vi "read_params.vi"(8 "error in (no error)":errorcluster caption="entrée d'erreur (pas d'erreur)", 11 "KMeans en entrée":refnum<class "KMeans.lvclass">) -> (0 "error out":errorcluster caption="sortie d'erreur", 2 "params":T1={"n_clusters"=8.0, "init"={"init_type"="k-means++", "init_list"=[]}, "n_init"=10.0, "max_iter"=300.0, "tol"=0.0001, "verbose"=0.0, "random_state"=0.0, "copy_x"=TRUE, "algorithm"="auto"}, 3 "KMeans en sortie":refnum<class "KMeans.lvclass">)   [LabVIEW 2020, in "KMeans.lvclass"]
uses:
  KMeans.lvclass
  Controls/kmeans_params.ctl
  KMeans.lvclass/KMeans.ctl
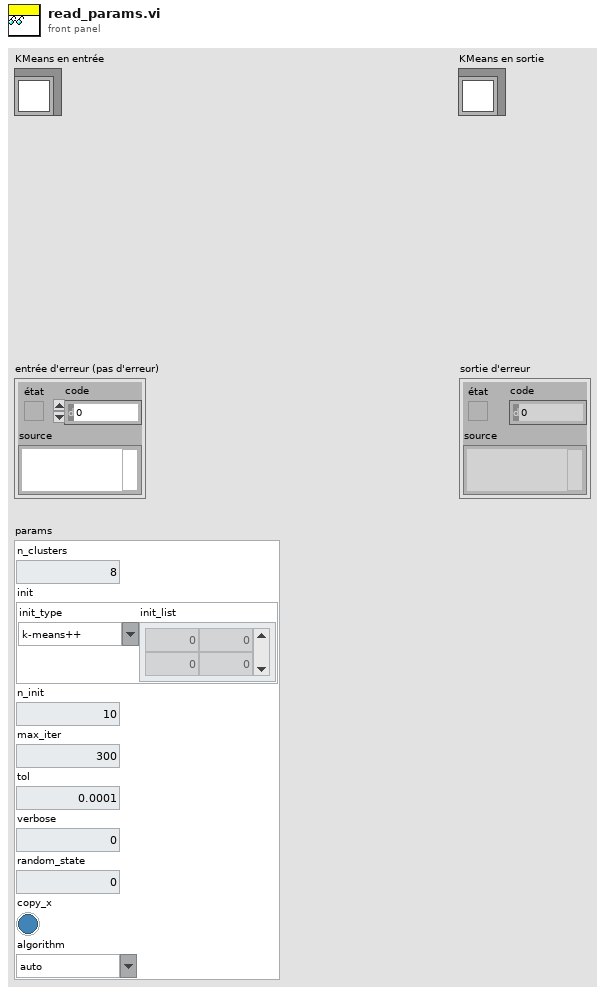
[diagram p1: front panel]
types:
  T1 = typedef "kmeans_params.ctl" = cluster{"n_clusters":dbl, "init":cluster{"init_type":string, "init_list":dbl[][]}, "n_init":dbl, "max_iter":dbl, "tol":dbl, "verbose":dbl, "random_state":dbl, "copy_x":bool, "algorithm":string}
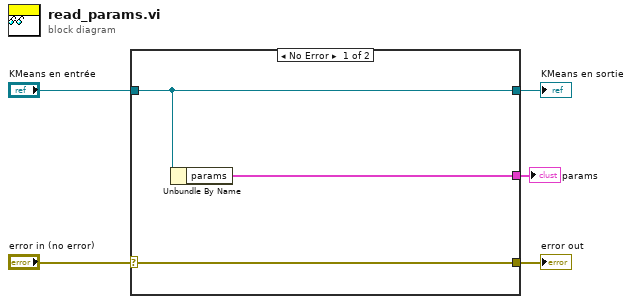
[diagram p0: block diagram]
diagram:
  n1 = case shown="No Error" "error in (no error)" {
    selector: "error in (no error)" -> [w8 w9]
    tunnel: [w8 w9] -> w4
    tunnel: [w7 w10] -> w2
    tunnel: "KMeans en entrée" -> [w7 w10]
    tunnel: [w6 _] -> w1
    frame No Error {
      n2 = Unbundle By Name(w7) -> ("params"=w6:T1)
    }
    frame Error {
    }
  }
  "error out" <- w4
  "KMeans en sortie" <- w2
  "params" <- w1
